vi "First Step.vi"(8 "error in (no error)":errorcluster, 11 "Pulse Gen Scan.lvclass in":refnum<class "Pulse Gen Scan.lvclass">) -> (0 "error out":errorcluster, 2 "Current Position":dbl, 3 "Pulse Gen Scan.lvclass out":refnum<class "Pulse Gen Scan.lvclass">)   [LabVIEW 2023, in "Pulse Gen Scan.lvclass"]
doc: "Goto step #0 - the first step. If desired, the scanner may do this in a different way than usual (i.e. by preparing to move a long distance, or reset to home position.)"
uses:
  Pulse Gen Scan.lvclass
  Pulse Gen Scan.lvclass/Pulse Gen Scan.ctl
  Scanner/Scanner.lvclass
panel:
  out "Array of Ch2 times used":dbl[unit][](array[numeric])
  out "Ch 1 Digital Waveform Graph":digitalwaveform(graph)
  out "Ch1 output string":string
  out "Ch2 output string":string
  out "Ch 2 Digital Waveform Graph":digitalwaveform(graph)
  out "Array of Ch1 times used":dbl[unit][](array[numeric])
  out "time per bit":dbl[unit]
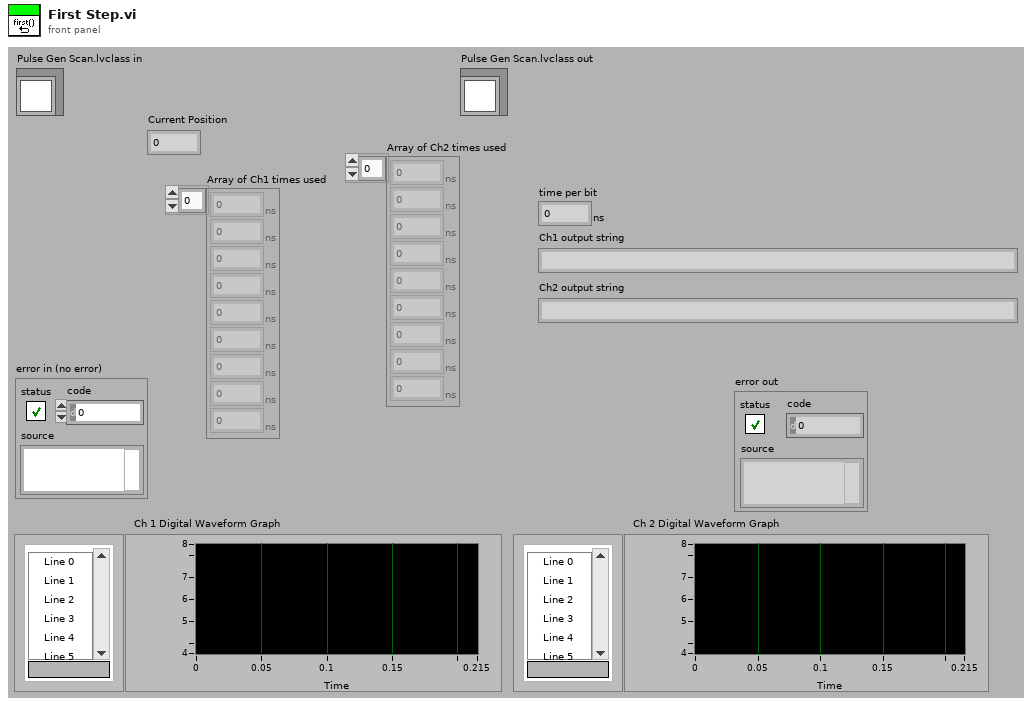
[diagram p1: front panel]
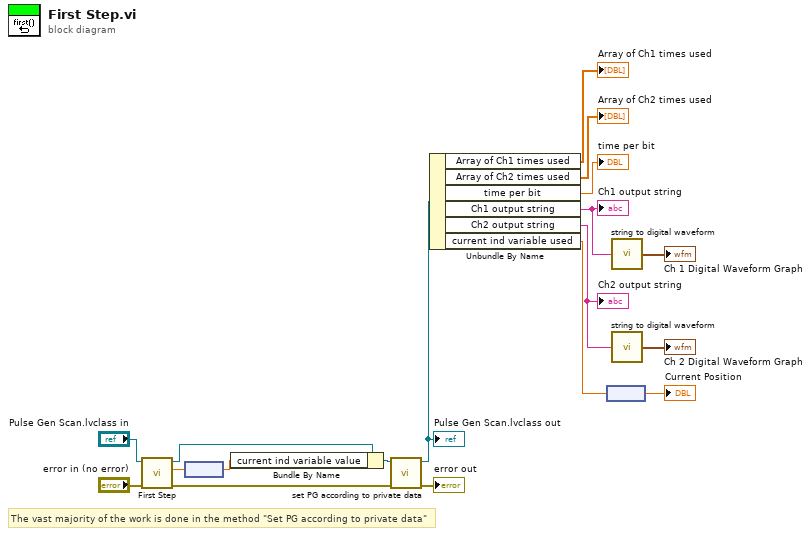
[diagram p0: block diagram]
diagram:
  # "The vast majority of the work is done in the method \"Set PG according to private data\""
  n1 = call-parent "First Step.vi"("error in (no error)"="error in (no error)", "Scanner.lvclass in"="Pulse Gen Scan.lvclass in") -> ("error out"=w1:errorcluster, "Current Position"=w12:dbl, "Scanner.lvclass out"=w13:refnum<class "Pulse Gen Scan.lvclass">)  [unwired: 7 out]
  n2 = node(w12) -> (w11:dbl[unit])
  n3 = Bundle By Name(cluster=w13, "current ind variable value"=w11) -> (w2:refnum<class "Pulse Gen Scan.lvclass">)
  n4 = call "set PG according to private data.vi"("error in (no error)"=w1, "Pulse Gen Scan in"=w2) -> ("error out"=→"error out":errorcluster, "Pulse Gen Scan out"=w9:refnum<class "Pulse Gen Scan.lvclass">)  [unwired: 8 out]
  "Pulse Gen Scan.lvclass out" <- w9
  n5 = Unbundle By Name(w9) -> ("Array of Ch1 times used"=→"Array of Ch1 times used":dbl[unit][], "Array of Ch2 times used"=→"Array of Ch2 times used":dbl[unit][], "time per bit"=→"time per bit":dbl[unit], "Ch1 output string"=w4:string, "Ch2 output string"=w3:string, "current ind variable used"=w8:dbl[unit])
  "Ch1 output string" <- w4
  "Ch2 output string" <- w3
  n6 = node(w8) -> (→"Current Position":dbl)
  n7 = call "string to digital waveform.vi"("String"=w4) -> ("digital waveform"=→"Ch 1 Digital Waveform Graph":digitalwaveform)
  n8 = call "string to digital waveform.vi"("String"=w3) -> ("digital waveform"=→"Ch 2 Digital Waveform Graph":digitalwaveform)
